vi "Create Instrument Addon Node.vi"(8 "Error In":errorcluster, 11 "Target In":refnum<k24>) -> (0 "Error Out":errorcluster, 2 "Instrument Addon Refnum":T1=18446744073709551615 format="%.0x", 3 "Target Out":refnum<k24>)   [LabVIEW 2018, in "Instrument Addon Scripting API.lvlib"]
uses:
  Instrument Addon Scripting API.lvlib
  NationalInstruments.VeriStand.SystemDefinitionAPI
  <vilib>/NI Veristand/Custom Device API/Custom Device Item Ref.ctl
  Addon/Addon Shared/SubVIs/Constants.vi
  Addon/Addon Shared/Instrument Addon Shared.lvlib
  <vilib>/NI Veristand/Custom Device Tools/Custom Device Utility Library/Custom Device Utility Library.lvlib
  <vilib>/NI Veristand/Custom Device API/Custom Device API.lvlib
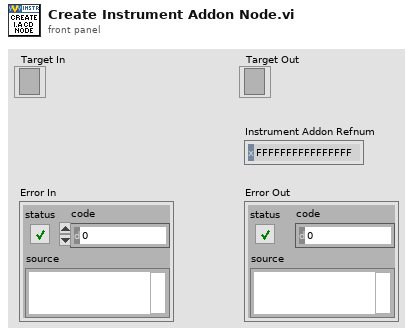
[diagram p1: front panel]
types:
  T1 = typedef "Custom Device API.lvlib/Custom Device Item Ref.ctl" = u64
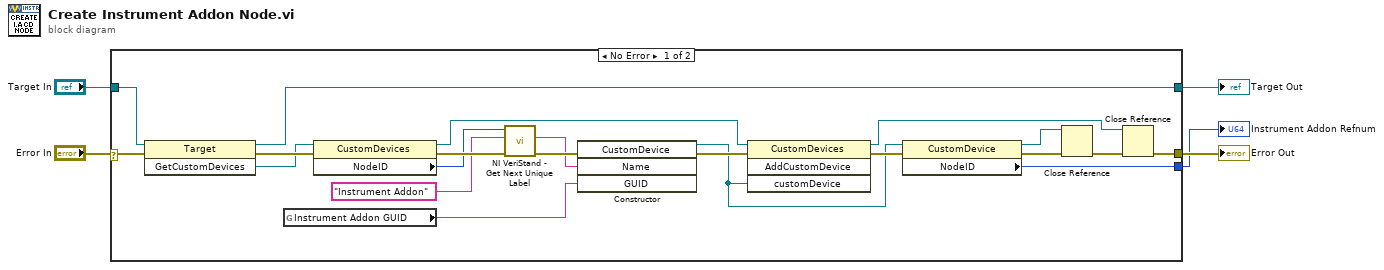
[diagram p0: block diagram]
diagram:
  n1 = case shown="No Error" "Error In" {
    selector: "Error In" -> [w10 w28]
    tunnel: [w26 _] -> w1
    tunnel: "Target In" -> [w25 w27]
    tunnel: [w8 w28] -> w3
    tunnel: [w6 w27] -> w2
    frame No Error {
      n2 = invoke class="Target" method="GetCustomDevices"(reference=w25, error in=w10) -> (reference out=w6:refnum<k24>, error out=w18:errorcluster, "GetCustomDevices"=w17:refnum<k24>)  [unwired: 1 in]
      n3 = global read "Constants.vi" "Instrument Addon GUID"() -> (w16:string)
      n4 = property class="CustomDevices"(reference=w17, error in=w18) -> (reference out=w21:refnum<k24>, error out=w23:errorcluster, "NodeID"=w19:u64)
      n5 = call <vilib>:"NI VeriStand - Get Next Unique Label.vi"("error in (no error)"=w23, "Label"="Instrument Addon" ("Name"), "Parent Ref in"=w19) -> ("error out"=w24:errorcluster, "Label out"=w22:string)  [unwired: 5 in, 2 out]
      n6 = constructor class="CustomDevice"(error in=w24, "Name"=w22, "GUID"=w16) -> (reference out=w13:refnum<k24>, error out=w15:errorcluster)  [unwired: 2 in, 3 out]
      n7 = invoke class="CustomDevices" method="AddCustomDevice"(reference=w21, error in=w15, "customDevice"=w13) -> (reference out=w7:refnum<k24>, error out=w14:errorcluster)  [unwired: 1 in, 2 out]
      n8 = property class="CustomDevice"(reference=w13, error in=w14) -> (reference out=w12:refnum<k24>, error out=w11:errorcluster, "NodeID"=w26:u64)
      n9 = Close Reference(reference=w12, error in (no error)=w11) -> (error out=w9:errorcluster)
      n10 = Close Reference(reference=w7, error in (no error)=w9) -> (error out=w8:errorcluster)
    }
    frame Error {
    }
  }
  "Error Out" <- w3
  "Target Out" <- w2
  "Instrument Addon Refnum" <- w1
